vi "Get Action Paths.vi"() -> (0 "paths":path[](array[path]))   [LabVIEW 2019]
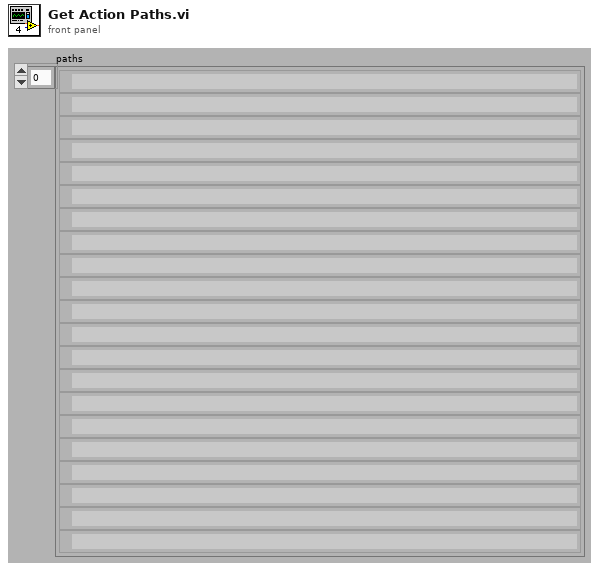
[diagram p1: front panel]
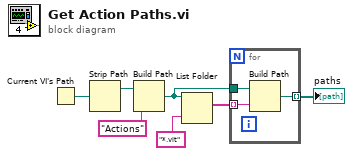
[diagram p0: block diagram]
diagram:
  n1 = Current VI's Path() -> (path=w4:path)
  n2 = Strip Path(path=w4) -> (stripped path=w5:path)  [unwired: 1 out]
  n3 = Build Path(base path=w5, name or relative path="Actions") -> (appended path=w3:path)
  n4 = List Folder(path=w3, pattern="*.vit") -> (filenames=w2:string[])  [unwired: 2 in, 3 out]
  n5 = for {
    tunnel: [w10] -> w1 mode=indexing
    tunnel: w3 -> [w9]
    tunnel: w2 -> [w8] mode=indexing
    n6 = Build Path(base path=w9, name or relative path=w8) -> (appended path=w10:path)
  }
  "paths" <- w1
